vi "saveMessages.vi"(8 "error in (no error)":errorcluster, 10 "FileName (without extension)":string="messages", 11 "simonMessages in":refnum<class "simonMessages.lvclass">) -> (0 "error out":errorcluster, 3 "simonMessages out":refnum<class "simonMessages.lvclass">)   [LabVIEW 2020, in "simonMessages.lvclass"]
uses:
  simonMessages.lvclass
  simonMessages.lvclass/simonMessages.ctl
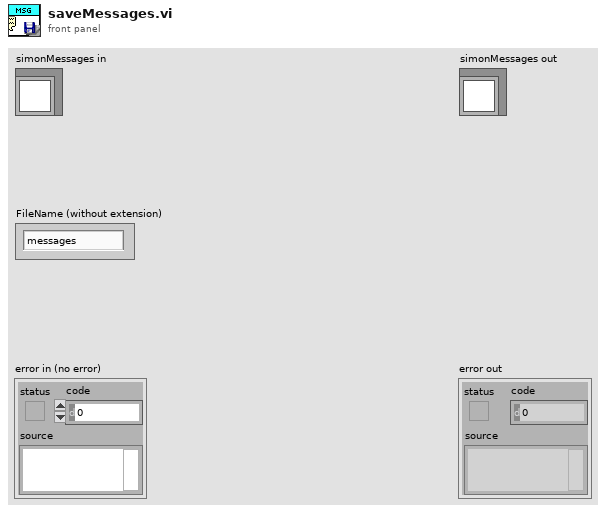
[diagram p1: front panel]
types:
  T1 = enum16{"open", "replace", "create", "open or create", "replace or create", "replace or create with confirmation"}
  T2 = map{string, cluster{"Text":string, "Size":u8, "Justification":enum16{"Left", "Center", "Right"}, "Display Type":string}}
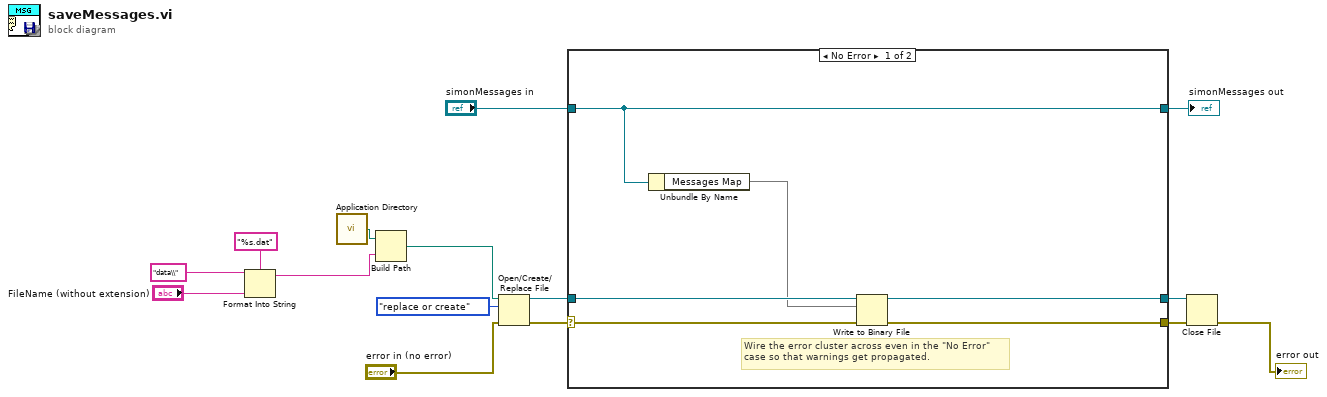
[diagram p0: block diagram]
diagram:
  n1 = Format Into String(format string="%s.dat" ("name or relative path"), initial string="data\\" ("name or relative path"), "FileName (without extension)") -> (resulting string=w2:string)  [unwired: 1 in, 1 out]
  n2 = call <vilib>:"Application Directory.vi"() -> ("Application Directory"=w13:path)
  n3 = Build Path(base path=w13, name or relative path=w2) -> (appended path=w12:path)
  n4 = Open/Create/Replace File(file path (use dialog)=w12, error in="error in (no error)", operation (0:open)=T1."replace or create") -> (refnum out=w10:refnum<file>, error out=w9:errorcluster)  [unwired: 3 in, 1 out]
  n5 = case shown="No Error" w9 {
    selector: w9 -> [w19 w23]
    tunnel: [w21 w24] -> w14
    tunnel: "simonMessages in" -> [w21 w24]
    tunnel: w10 -> [w20 w22]
    tunnel: [w17 w22] -> w8
    tunnel: [w16 w23] -> w7
    frame No Error {
      # "Wire the error cluster across even in the \"No Error\"\ncase so that warnings get propagated."
      n6 = Unbundle By Name(w21) -> ("Messages Map"=w18:T2)
      n7 = Write to Binary File(file (use dialog)=w20, data=w18, error in=w19) -> (refnum out=w17:refnum<file>, error out=w16:errorcluster)  [unwired: 3 in, 1 out]
    }
    frame Error {
    }
  }
  "simonMessages out" <- w14
  n8 = Close File(refnum=w8, error in=w7) -> (error out=→"error out":errorcluster)  [unwired: 1 out]
